vi "AVS_excitation.vi"(2 "AVS-Temperatur":dbl, 3 "Pfad":path) -> (1 "Excitation AVS":dbl)   [LabVIEW 2019]
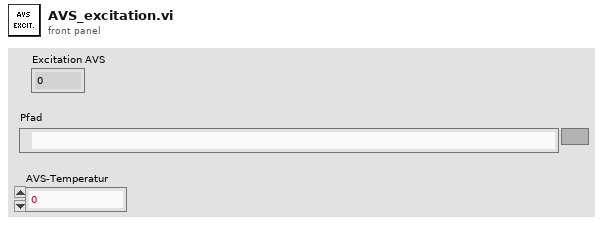
[diagram p1: front panel]
types:
  T1 = enum16{"open", "replace", "create", "open or create", "replace or create", "replace or create with confirmation"}
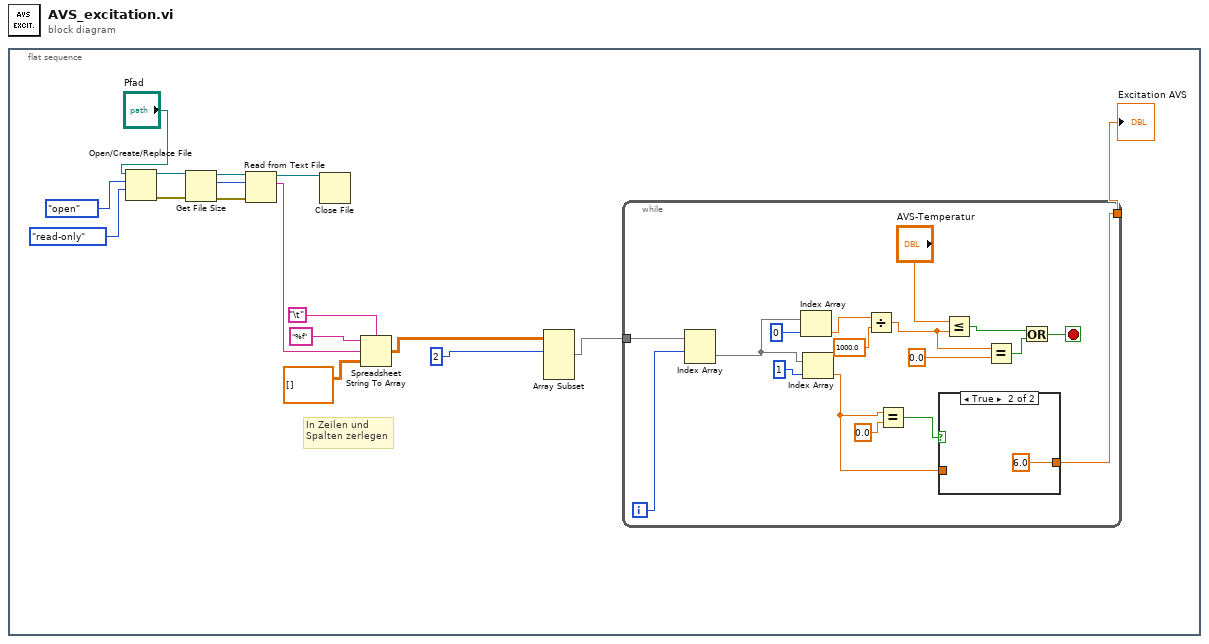
[diagram p0: block diagram]
diagram:
  n1 = flat-sequence {
    frame #0 {
      # "In Zeilen und \nSpalten zerlegen"
      n2 = Open/Create/Replace File(file path (use dialog)="Pfad", operation (0:open)=T1."open", access (0:read/write)=enum16{"read/write", "read-only", "write-only"}."read-only") -> (refnum out=w14:refnum<file>, error out=w11:errorcluster)  [unwired: 3 in, 1 out]
      n3 = Get File Size(file=w14, error in=w11) -> (refnum out=w13:refnum<file>, size (in bytes)=w9:i64, 0:w10:errorcluster)
      n4 = Read from Text File(file (use dialog)=w13, count=w9, error in=w10) -> (refnum out=w12:refnum<file>, text=w5:string)  [unwired: 1 in, 2 out]
      n5 = Close File(refnum=w12) -> ()  [unwired: 1 in, 2 out]
      n6 = Spreadsheet String To Array(delimiter (Tab)="\t", format string="%f", spreadsheet string=w5, array type (2D Dbl)=dbl[][] []) -> (array=w3:dbl[][])
      n7 = Array Subset(array=w3, index (row)=2) -> (w2:dbl[][])  [unwired: 3 in]
      n8 = while {
        tunnel: w2 -> [w33]
        tunnel: [w18] -> w1
        i -> [w34]
        stop <- w24 stop-if-true
        n9 = Index Array(array=w33, index (row)=w34) -> (element=w30:dbl[])  [unwired: 1 in]
        n10 = Index Array(array=w30, index=0) -> (element=w28:dbl)
        n11 = Index Array(array=w30, index=1) -> (element=w21:dbl)
        n12 = Divide(x=w28, y=1000.0) -> (x/y=w26:dbl)
        n13 = Equal?(x=w21, y=0.0) -> (x = y?=w19:bool)
        n14 = case shown="True" w19 {
          tunnel: w21 -> [w35 _]
          tunnel: [w35 6.0] -> w18
          frame False {
          }
          frame True {
          }
        }
        n15 = Less Or Equal?(x="AVS-Temperatur", y=w26) -> (x <= y?=w23:bool)
        n16 = Equal?(x=w26, y=0.0) -> (x = y?=w22:bool)
        n17 = Or(x=w23, y=w22) -> (x .or. y?=w24:bool)
      }
      "Excitation AVS" <- w1
    }
  }
